vi "Fake Recreate Client.vi"(8 "error in":errorcluster, 10 "cluster id":string, 11 "grpc client id in":T1) -> (0 "error out":errorcluster, 3 "grpc client id out":T1)   [LabVIEW 2020, in "MeasurementServerTests.lvlib" / "Discovery Tests.lvlib"]
uses:
  Discovery Tests.lvlib
  <vilib>/gRPC/LabVIEW gRPC Library/Shared/grpcId.ctl
  <vilib>/gRPC/LabVIEW gRPC Library/grpc-lvsupport-release.lvlib
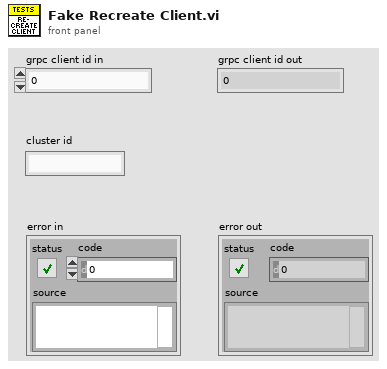
[diagram p1: front panel]
types:
  T1 = typedef "grpc-lvsupport-release.lvlib/grpcId.ctl" = u64
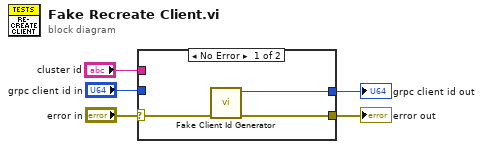
[diagram p0: block diagram]
diagram:
  n1 = case shown="No Error" "error in" {
    selector: "error in" -> [w8 w9]
    tunnel: [w7 w9] -> w4
    tunnel: [w6 _] -> w3
    tunnel: "grpc client id in" -> [_ _]
    tunnel: "cluster id" -> [_ _]
    frame No Error {
      n2 = call "Fake Client Id Generator.vi"("error in"=w8) -> ("error out"=w7:errorcluster, "client id"=w6:u64)  [unwired: 9 in]
    }
    frame Error {
    }
  }
  "error out" <- w4
  "grpc client id out" <- w3
